vi "main.vi"(8 "error in":errorcluster) -> (0 "error out":errorcluster)   [LabVIEW 2018, in "Error Handler.lvlib"]
uses:
  Error Handler.lvlib
  Common/Common.lvlib
  Common/vi/Stop All - Action.ctl
  ctl/Queue Actions.ctl
  ctl/Module State.ctl
  ctl/Error Type.ctl
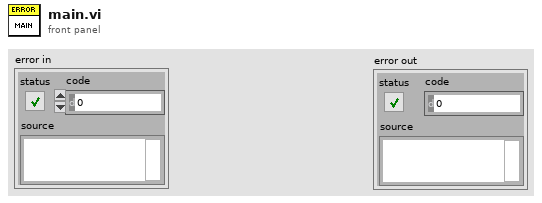
[diagram p1: front panel]
types:
  T1 = typedef "Error Handler.lvlib/Error Type.ctl" = enum16{"Minor Error", "Wash Cycle Error", "System Error"}
  T2 = cluster{"Error Type":T1, "Description":string, "Station and step":string}
  T3 = typedef "Error Handler.lvlib/Module State.ctl" = enum16{"Init", "Idle", "Error", "Close", "Handle External Error", "Log Error"}
  T4 = typedef "Error Handler.lvlib/Queue Actions.ctl" = enum16{"Create", "Get", "Destroy"}
  T5 = typedef "Common.lvlib/Stop All - Action.ctl" = enum16{"Create", "Get", "Fire", "Destroy"}
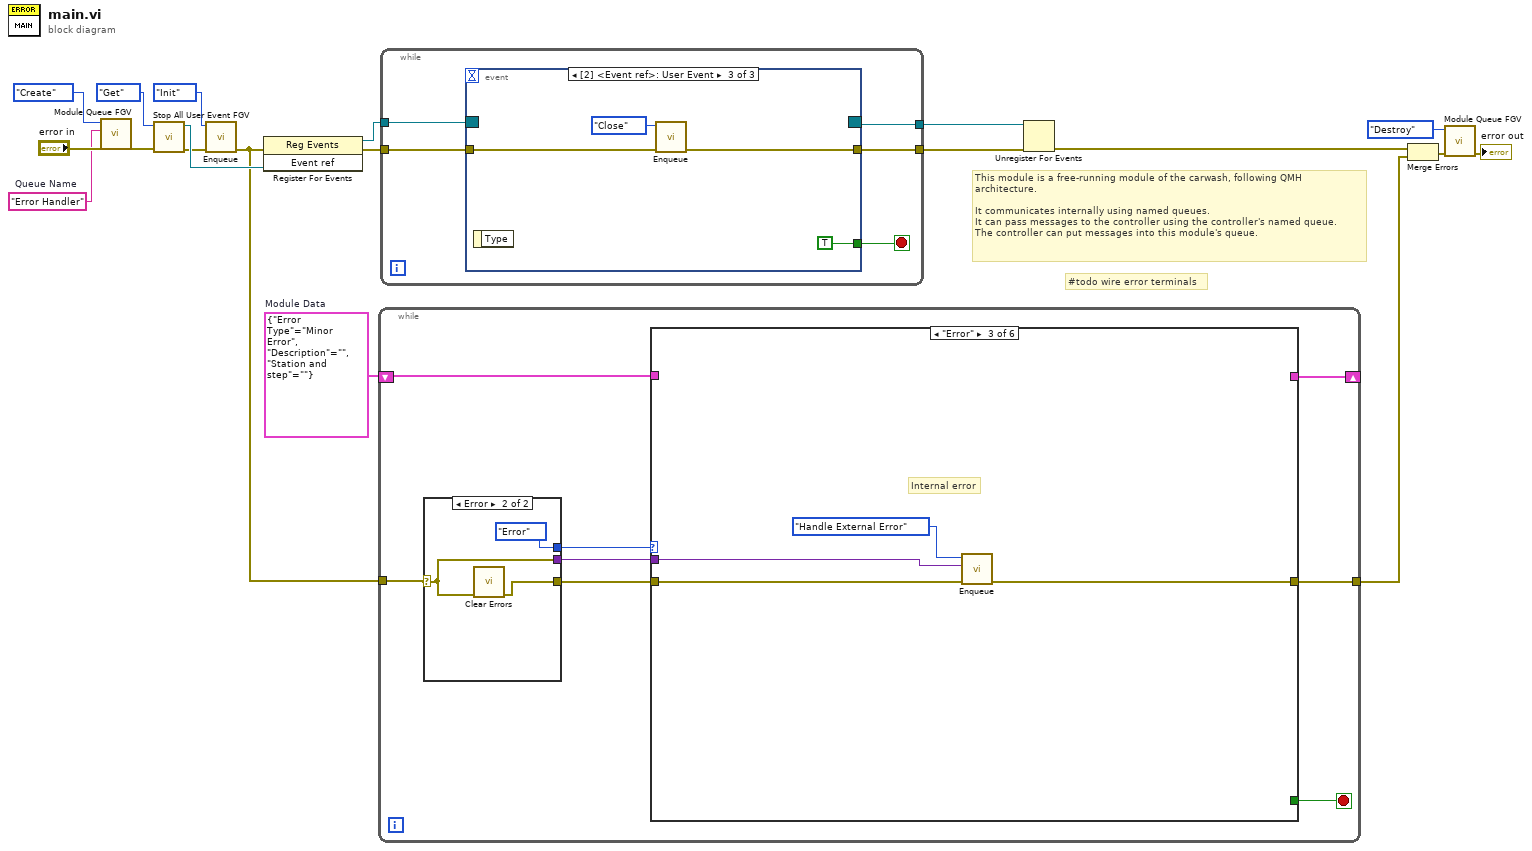
[diagram p0: block diagram]
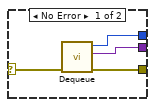
[diagram p2: hidden frame]
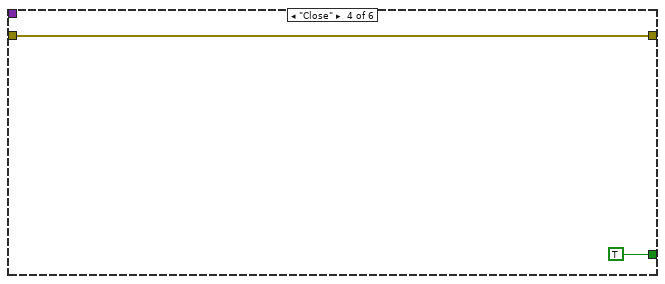
[diagram p5: hidden frame]
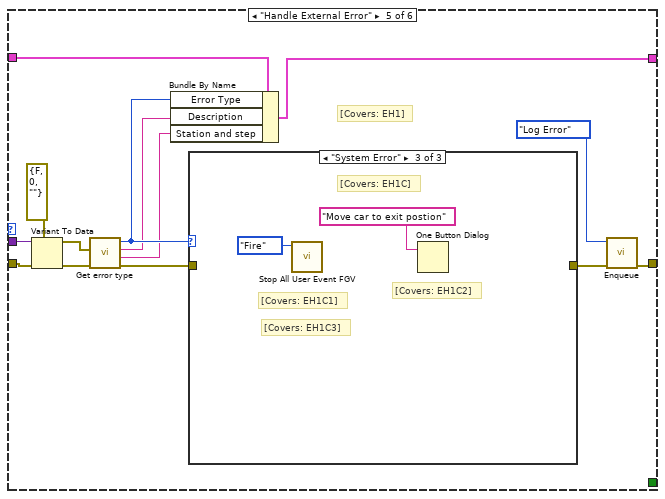
[diagram p6: hidden frame]
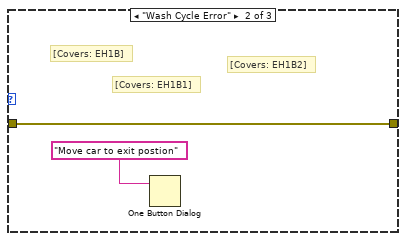
[diagram p8: hidden frame]
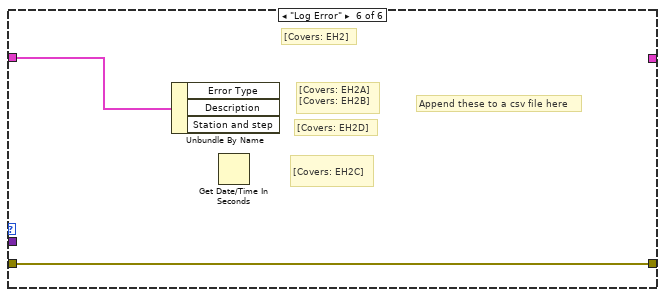
[diagram p9: hidden frame]
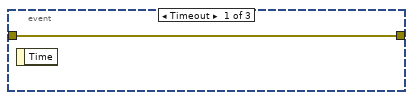
[diagram p10: hidden frame]
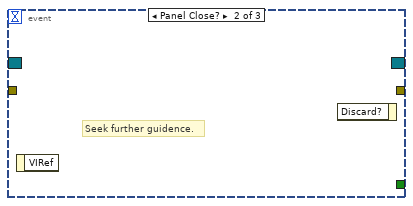
[diagram p11: hidden frame]
diagram:
  w2 = "Error Handler"  # Queue Name
  w1 = T2 {"Error Type"=enum."Minor Error", "Description"="", "Station and step"=""}  # Module Data
  # "#todo wire error terminals"
  # "This module is a free-running module of the carwash, following QMH\narchitecture.\n\nIt communicates internally using named queues.\nIt can pass messages to the controller using the controller's named queue.\nThe controller can put messages into this module's queue."
  n1 = call "Module Queue FGV.vi"("error in"="error in", "Queue Name"=w2, "Action"=Queue_Actions."Create") -> ("error out"=w16:errorcluster)  [unwired: 7 in, 1 out]
  n2 = call "Stop All User Event FGV.vi"("error in"=w16, "Action"=Stop_All_-_Action."Get") -> ("error out"=w15:errorcluster, "Event ref"=w18:refnum<user-event>)  [unwired: 8 in]
  n3 = call "Enqueue.vi"("error in"=w15, "State"=Module_State."Init") -> ("error out"=w7:errorcluster)  [unwired: 9 in]
  n4 = register-events(error in=w7, w18) -> (reference out=w13:refnum<event-registration>, error out=w11:errorcluster)  [unwired: 1 in]
  n5 = while {
    tunnel: w7 -> [w27]
    tunnel: [w22] -> w6
    shift-right: [w20] -> _
    shift-left: w1 -> [w21]
    stop <- w23 stop-if-true
    n6 = case shown="Error" w27 {
      selector: w27 -> [w31 w33]
      tunnel: [w30 w32] -> w24
      tunnel: [w29 w33] -> w25
      tunnel: [w28 Module_State."Error" ("State")] -> w26
      frame No Error {
        n7 = call "Dequeue.vi"("error in"=w31) -> ("error out"=w30:errorcluster, "Data"=w29:variant, "State"=w28:T3)  [unwired: 8 in]
      }
      frame Error {
        n8 = call <vilib>:"Clear Errors.vi"("error in (no error)"=w33) -> ("error out"=w32:errorcluster)  [unwired: 5 in, 1 out]
      }
    }
    n9 = case shown="\"Error\"" w26 {
      tunnel: w25 -> [_ _ w37 _ w43 _]
      tunnel: w24 -> [_ _ w35 w39 w50 w59]
      tunnel: [_ _ _ TRUE _ _] -> w23
      tunnel: [_ _ w36 w39 w45 w59] -> w22
      tunnel: w21 -> [_ _ _ _ w52 w60]
      tunnel: [_ _ _ _ w53 _] -> w20
      frame "Init", Default {
      }
      frame "Idle" {
      }
      frame "Error" {
        # "Internal error"
        n10 = call "Enqueue.vi"("error in"=w35, "Data"=w37, "State"=Module_State."Handle External Error") -> ("error out"=w36:errorcluster)  [unwired: 8 in]
      }
      frame "Close" {
      }
      frame "Handle External Error" {
        # "[Covers: EH1]"
        n11 = Variant To Data(error in=w50, type=errorcluster {"status"=FALSE, "code"=0, "source"=""} ("error constant"), Variant=w43) -> (data=w42:errorcluster, error out=w54:errorcluster)
        n12 = call "Get error type.vi"("error in"=w54, "error to look up"=w42) -> ("error out"=w51:errorcluster, "Station and step"=w41:string, "Description"=w48:string, "Error Type"=w49:T1)  [unwired: 6 in]
        n13 = Bundle By Name(cluster=w52, "Error Type"=w49, "Description"=w48, "Station and step"=w41) -> (w53:T2)
        n14 = case shown="\"System Error\"" w49 {
          tunnel: [_ w56 _] -> w46
          tunnel: w51 -> [_ w56 _]
          frame "Minor Error", Default {
            # "Do nothing"
            # "[Covers: EH1A]"
          }
          frame "Wash Cycle Error" {
            # "[Covers: EH1B2]"
            # "[Covers: EH1B1]"
            # "[Covers: EH1B]"
            n15 = One Button Dialog(message="Move car to exit postion") -> ()  [unwired: 1 in, 1 out]
          }
          frame "System Error" {
            # "[Covers: EH1C3]"
            # "[Covers: EH1C2]"
            # "[Covers: EH1C1]"
            # "[Covers: EH1C]"
            n16 = call "Stop All User Event FGV.vi"("Action"=Stop_All_-_Action."Fire") -> ()  [unwired: 9 in, 2 out]
            n17 = One Button Dialog(message="Move car to exit postion") -> ()  [unwired: 1 in, 1 out]
          }
        }
        n18 = call "Enqueue.vi"("error in"=w46, "State"=Module_State."Log Error") -> ("error out"=w45:errorcluster)  [unwired: 9 in]
      }
      frame "Log Error" {
        # "[Covers: EH2C]"
        # "[Covers: EH2D]"
        # "[Covers: EH2A]\n[Covers: EH2B]"
        # "[Covers: EH2]"
        # "Append these to a csv file here"
        n19 = Unbundle By Name(w60) -> ()  [unwired: 3 out]
        n20 = Get Date/Time In Seconds() -> ()  [unwired: 1 out]
      }
    }
  }
  n21 = while {
    tunnel: w13 -> [w65]
    tunnel: [w64] -> w12
    tunnel: [w63] -> w10
    tunnel: w11 -> [w62]
    stop <- w61 stop-if-true
    n22 = event shown="[2] <Event ref>: User Event" {
      selector: w65 -> [_ _ _]
      dyn-events: [_ _ _] -> w64
      timeout: _ -> [_ _ _]
      tunnel: [w66 _ w69] -> w63
      tunnel: w62 -> [w66 _ w70]
      tunnel: [_ _ TRUE] -> w61
      event Timeout {
        n23 = event-data() -> ()  [unwired: 1 in, 1 out]
      }
      event Panel Close? {
        # "Seek further guidence."
        n24 = event-data() -> ()  [unwired: 1 in, 1 out]
        n25 = event-data() -> ()  [unwired: 2 in, 1 out]
      }
      event User Event {
        n26 = event-data() -> ()  [unwired: 1 in, 1 out]
        n27 = call "Enqueue.vi"("error in"=w70, "State"=Module_State."Close") -> ("error out"=w69:errorcluster)  [unwired: 9 in]
      }
    }
  }
  n28 = Unregister For Events(event registration refnum=w12, error in=w10) -> (error out=w3:errorcluster)
  n29 = Merge Errors(w3, w6) -> (w5:errorcluster)
  n30 = call "Module Queue FGV.vi"("error in"=w5, "Action"=Queue_Actions."Destroy") -> ("error out"=→"error out":errorcluster)  [unwired: 8 in, 1 out]
